vi "FuseTargeting.vi"(0 "Estimated Distance to Target (in)":dbl, 1 "Estimated Heading to Target (deg)":dbl, 7 "LIDAR Distance to Target (in)":dbl, 9 "LimeLight Distance to Target (in)":dbl, 11 "LimeLight Heading to Target (deg)":dbl, 13 "Robot_H (deg)":dbl) -> (14 "Fused Distance to Target (in)":dbl, 15 "Fused Heading to Target (deg)":dbl, 16 "Fused Heading to Target Delta (deg)":dbl, 17 "Pointed at Target":bool)   [LabVIEW 2020]
doc: "This VI fuses data from multiple sensing modalities to estimate the robot's range and heading-error to the target."
uses:
  driverdata.vi
  sensordata.vi
panel:
  in  "Loops to Average Distance":i32=15
  in  "Min Timed Aligned (ms)":u32=500
  in  "Acceptable Heading Error (deg)":dbl=4.0
  in  "Loops to Average Heading":i32=15
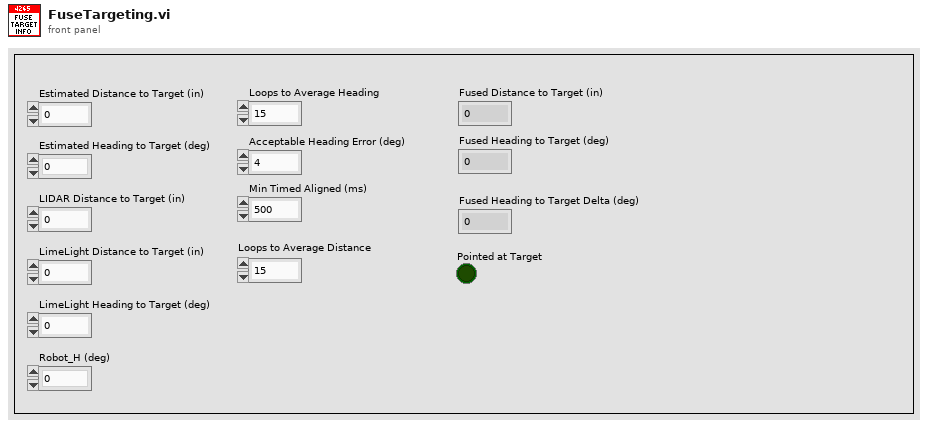
[diagram p1: front panel]
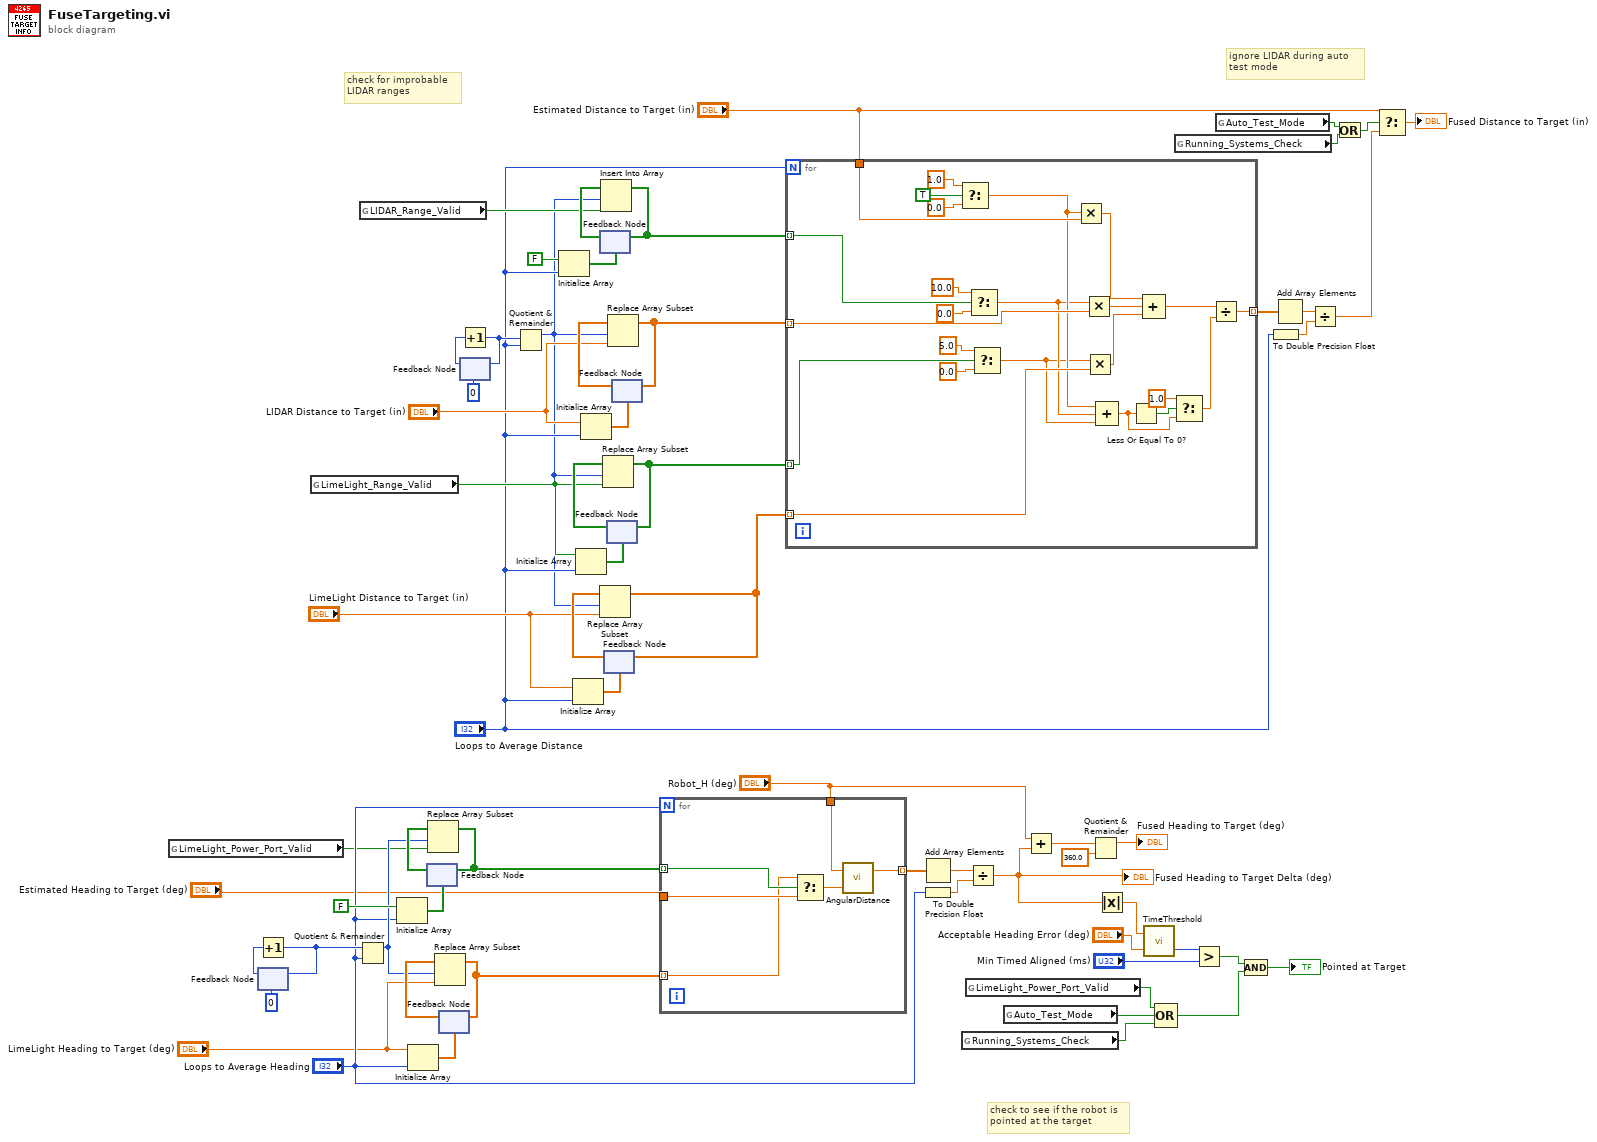
[diagram p0: block diagram]
diagram:
  # "check for improbable\nLIDAR ranges"
  # "check to see if the robot is\npointed at the target"
  # "ignore LIDAR during auto\ntest mode"
  n1 = global read "sensordata.vi" "LimeLight_Power_Port_Valid"() -> (w27:bool)
  n2 = feedback #1(0) -> (w61:i32)
  n3 = Increment(x=w61) -> (x+1=w60:i32)
  n4 = feedback-in #1(w60) -> ()
  n5 = global read "sensordata.vi" "LimeLight_Range_Valid"() -> (w17:bool)
  n6 = Quotient & Remainder(x=w60, y="Loops to Average Heading") -> (x-y*floor(x/y)=w55:i32)  [unwired: 1 out]
  n7 = global read "sensordata.vi" "LIDAR_Range_Valid"() -> (w20:bool)
  n8 = Initialize Array(FALSE, "Loops to Average Heading") -> (w57:bool[])
  n9 = Initialize Array("LimeLight Heading to Target (deg)", "Loops to Average Heading") -> (w64:dbl[])
  n10 = feedback #2(w57) -> (w59:bool[])
  n11 = Replace Array Subset(array=w59, new element=w27, index=w55) -> (w56:bool[])
  n12 = feedback-in #2(w56) -> ()
  n13 = feedback #3(w64) -> (w63:dbl[])
  n14 = Replace Array Subset(array=w63, new element="LimeLight Heading to Target (deg)", index=w55) -> (w26:dbl[])
  n15 = feedback-in #3(w26) -> ()
  n16 = feedback #4(0) -> (w30:i32)
  n17 = Increment(x=w30) -> (x+1=w29:i32)
  n18 = feedback-in #4(w29) -> ()
  n19 = Quotient & Remainder(x=w29, y="Loops to Average Distance") -> (x-y*floor(x/y)=w11:i32)  [unwired: 1 out]
  n20 = Initialize Array(FALSE, "Loops to Average Distance") -> (w39:bool[])
  n21 = Initialize Array("LimeLight Distance to Target (in)", "Loops to Average Distance") -> (w14:dbl[])
  n22 = Initialize Array(w17, "Loops to Average Distance") -> (w19:bool[])
  n23 = Initialize Array("LIDAR Distance to Target (in)", "Loops to Average Distance") -> (w43:dbl[])
  n24 = feedback #5(w39) -> (w41:bool[])
  n25 = Insert Into Array(array=w41, index=w11, new element=w20) -> (w38:bool[])
  n26 = feedback-in #5(w38) -> ()
  n27 = feedback #6(w14) -> (w15:dbl[])
  n28 = Replace Array Subset(array=w15, new element="LimeLight Distance to Target (in)", index=w11) -> (w10:dbl[])
  n29 = feedback-in #6(w10) -> ()
  n30 = feedback #7(w19) -> (w18:bool[])
  n31 = Replace Array Subset(array=w18, new element=w17, index=w11) -> (w16:bool[])
  n32 = feedback-in #7(w16) -> ()
  n33 = feedback #8(w43) -> (w42:dbl[])
  n34 = Replace Array Subset(array=w42, new element="LIDAR Distance to Target (in)", index=w11) -> (w37:dbl[])
  n35 = feedback-in #8(w37) -> ()
  n36 = for {
    N: "Loops to Average Heading" -> [_]
    tunnel: w56 -> [w70] mode=indexing
    tunnel: w26 -> [w65] mode=indexing
    tunnel: "Estimated Heading to Target (deg)" -> [w69]
    tunnel: "Robot_H (deg)" -> [w68]
    tunnel: [w66] -> w54 mode=indexing
    n37 = Select(t=w65, s=w70, f=w69) -> (s? t:f=w67:dbl)
    n38 = call "AngularDistance.vi"("Goal Angle (deg) [0,360]"=w67, "Current Angle (deg) [-Inf,+Inf]"=w68) -> ("Signed Angular Distance (deg) [-180,+180]"=w66:dbl)  [unwired: 1 out]
  }
  n39 = for {
    N: "Loops to Average Distance" -> [_]
    tunnel: w38 -> [w81] mode=indexing
    tunnel: w37 -> [w82] mode=indexing
    tunnel: w16 -> [w80] mode=indexing
    tunnel: w10 -> [w79] mode=indexing
    tunnel: "Estimated Distance to Target (in)" -> [w83]
    tunnel: [w78] -> w8 mode=indexing
    n40 = Select(t=1.0, s=TRUE, f=0.0) -> (s? t:f=w77:dbl)
    n41 = Select(t=10.0, s=w81, f=0.0) -> (s? t:f=w76:dbl)
    n42 = Select(t=5.0, s=w80, f=0.0) -> (s? t:f=w75:dbl)
    n43 = Multiply(x=w77, y=w83) -> (x*y=w89:dbl)
    n44 = Multiply(x=w76, y=w82) -> (x*y=w88:dbl)
    n45 = Multiply(x=w75, y=w79) -> (x*y=w85:dbl)
    n46 = Compound Arithmetic op=ADD(w77, w76, w75) -> (w73:dbl)
    n47 = Less Or Equal To 0?(x=w73) -> (x <= 0?=w74:bool)
    n48 = Compound Arithmetic op=ADD(w89, w88, w85) -> (w94:dbl)
    n49 = Select(t=1.0, s=w74, f=w73) -> (s? t:f=w71:dbl)
    n50 = Divide(x=w94, y=w71) -> (x/y=w78:dbl)
  }
  n51 = Add Array Elements(numeric array=w54) -> (sum=w53:dbl)
  n52 = To Double Precision Float(number="Loops to Average Heading") -> (double precision float=w52:dbl)
  n53 = global read "driverdata.vi" "Running_Systems_Check"() -> (w4:bool)
  n54 = global read "sensordata.vi" "LimeLight_Power_Port_Valid"() -> (w6:bool)
  n55 = Divide(x=w53, y=w52) -> (x/y=w21:dbl)
  "Fused Heading to Target Delta (deg)" <- w21
  n56 = global read "driverdata.vi" "Auto_Test_Mode"() -> (w7:bool)
  n57 = Add(x="Robot_H (deg)", y=w21) -> (x+y=w25:dbl)
  n58 = Quotient & Remainder(x=w25, y=360.0) -> (x-y*floor(x/y)=→"Fused Heading to Target (deg)":dbl)  [unwired: 1 out]
  n59 = Absolute Value(x=w21) -> (abs(x)=w48:dbl)
  n60 = call "TimeThreshold.vi"("Threshold"="Acceptable Heading Error (deg)", "Current Value"=w48) -> ("Time Below Threshold (ms)"=w46:u32)  [unwired: 1 out]
  n61 = Compound Arithmetic op=OR(w6, w7, w4) -> (w5:bool)
  n62 = global read "driverdata.vi" "Running_Systems_Check"() -> (w2:bool)
  n63 = Greater?(x=w46, y="Min Timed Aligned (ms)") -> (0:w44:bool)
  n64 = global read "driverdata.vi" "Auto_Test_Mode"() -> (w3:bool)
  n65 = Compound Arithmetic op=AND(w44, w5) -> (→"Pointed at Target":bool)
  n66 = To Double Precision Float(number="Loops to Average Distance") -> (double precision float=w35:dbl)
  n67 = Add Array Elements(numeric array=w8) -> (sum=w36:dbl)
  n68 = Divide(x=w36, y=w35) -> (x/y=w34:dbl)
  n69 = Or(x=w3, y=w2) -> (x .or. y?=w1:bool)
  n70 = Select(t="Estimated Distance to Target (in)", s=w1, f=w34) -> (s? t:f=→"Fused Distance to Target (in)":dbl)
